vi "Get Size.vi"(8 "error in (no error)":errorcluster, 11 "Array in":refnum<class "Array.lvclass">) -> (0 "error out":errorcluster, 2 "Size out":i32, 3 "Array out":refnum<class "Array.lvclass">)   [LabVIEW 2013, in "MDSplus.lvlib" / "Array.lvclass"]
uses:
  <vilib>/MDSplus/Classes/Data_Class/Array_Class/Array.lvclass
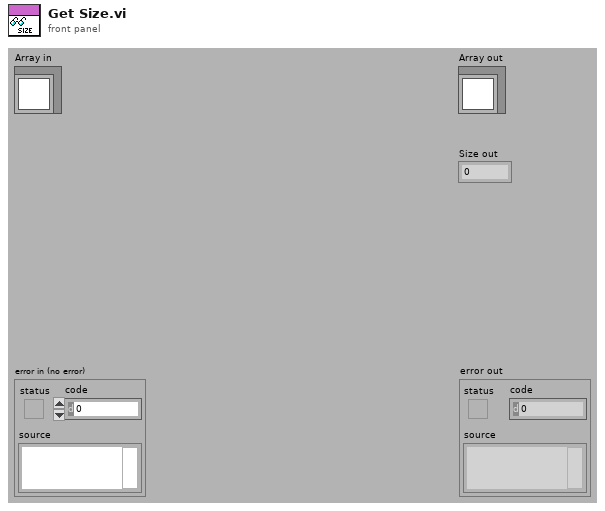
[diagram p1: front panel]
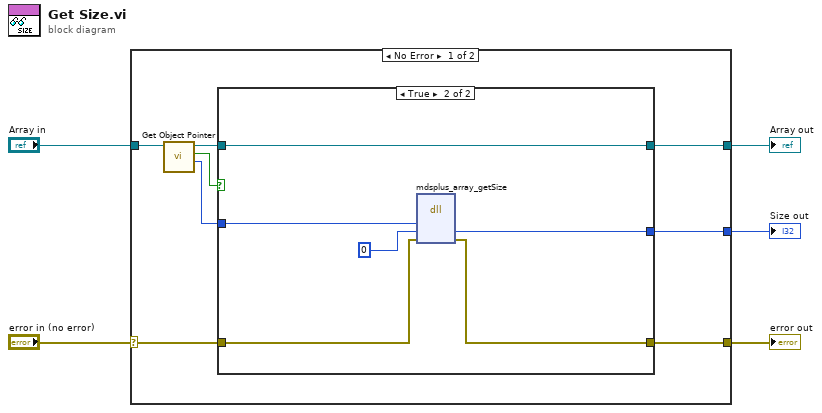
[diagram p0: block diagram]
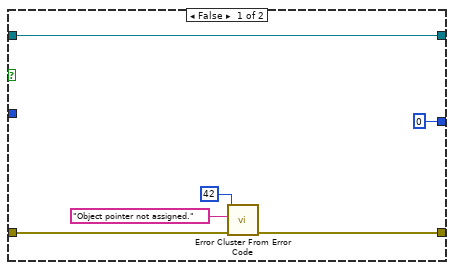
[diagram p2: hidden frame]
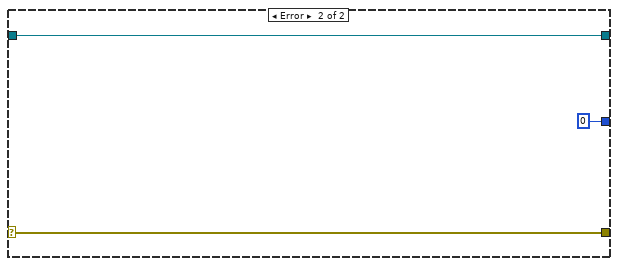
[diagram p3: hidden frame]
diagram:
  n1 = case shown="No Error" "error in (no error)" {
    selector: "error in (no error)" -> [w8 w28]
    tunnel: [w7 w28] -> w4
    tunnel: [w6 w27] -> w2
    tunnel: "Array in" -> [w13 w27]
    tunnel: [w12 0 ("lvFltArrHdlOut")] -> w1
    frame No Error {
      n2 = call-dynamic "Get Object Pointer.vi"("Data in"=w13) -> ("Object Pointer"=w10:i64, "Assigned object pointer?"=w11:bool, "Data out"=w9:refnum<class "Array.lvclass">)  [unwired: 8 in]
      n3 = case shown="True" w11 {
        tunnel: [0 ("lvFltArrHdlOut") w24] -> w12
        tunnel: w10 -> [_ w23]
        tunnel: w9 -> [w19 w20]
        tunnel: w8 -> [w15 w22]
        tunnel: [w14 w21] -> w7
        tunnel: [w19 w20] -> w6
        frame False {
          n4 = call <vilib>:"Error Cluster From Error Code.vi"("error in (no error)"=w15, "error message (\"\")"="Object pointer not assigned." ("error message (\"\")"), "error code (0)"=42) -> ("error out"=w14:errorcluster)  [unwired: 6 in]
        }
        frame True {
          n5 = dll-call lib="MDSobjectsLVShr" fn="mdsplus_array_getSize"("lvArrayPtr"=w23, "sizeOut"=0 ("floatOut"), "error"=w22) -> ("sizeOut"=w24:i32, "error"=w21:errorcluster)  [unwired: 5 in, 2 out]
        }
      }
    }
    frame Error {
    }
  }
  "error out" <- w4
  "Array out" <- w2
  "Size out" <- w1
